vi "ToRepo.vi"(8 "error in":errorcluster, 9 "to repo cluster":T1, 10 "repository in":refnum<class "NISE_CEF_Repository.lvclass">, 11 "node in":refnum<class "NISE_CEF_serializable node.lvclass">) -> (0 "error out":errorcluster, 2 "repository out":refnum<class "NISE_CEF_Repository.lvclass">, 3 "node out":refnum<class "NISE_CEF_serializable node.lvclass">)   [LabVIEW 2013, in "NISE_CEF_serializable node.lvclass"]
doc: "Transfers the information from the tree node into the repo. How it is stored in the repo depends on the Repo."
uses:
  NISE_CEF_serializable node.lvclass
  Repository/NISE_CEF_Repository.lvclass
  Node/ToRepoCluster.ctl
  hierarchy repo/NISE_CEF_HierarchyRepo.lvclass
  Node/NISE_CEF_Node.lvclass
  serializable configuration/NISE_CEF_serializable configuration.lvclass/NISE_CEF_serializable configuration.ctl
  serializable configuration/NISE_CEF_serializable configuration.lvclass
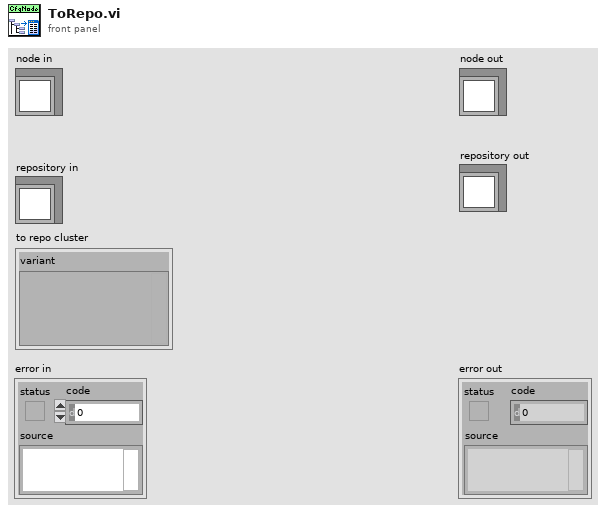
[diagram p1: front panel]
types:
  T1 = typedef "NISE_CEF_Node.lvclass/ToRepoCluster.ctl" = cluster{"variant":variant}
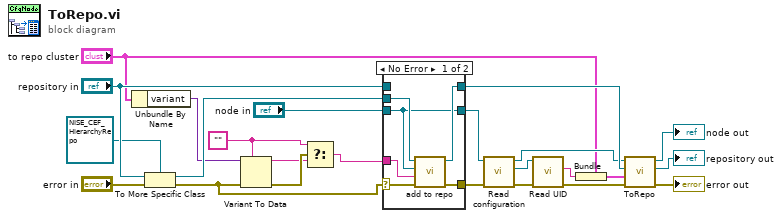
[diagram p0: block diagram]
diagram:
  w2 = ""
  n1 = Unbundle By Name("to repo cluster") -> ("variant"=w15:variant)
  n2 = To More Specific Class(target class=refnum<class "NISE_CEF_HierarchyRepo.lvclass"> refnum ("NISE_CEF_HierarchyRepo.lvclass"), reference="repository in", error in="error in") -> (specific class reference=w20:refnum<class "NISE_CEF_HierarchyRepo.lvclass">, error out=w5:errorcluster)
  n3 = Variant To Data(error in=w5, type=w2, Variant=w15) -> (data=w3:string, error out=w4:errorcluster)
  n4 = Select(t=w2, s=w4, f=w3) -> (s? t:f=w1:string)
  n5 = case shown="No Error" w5 {
    selector: w5 -> [w27 w32]
    tunnel: "repository in" -> [_ w33]
    tunnel: [w29 w33] -> w16
    tunnel: [w28 w32] -> w10
    tunnel: "node in" -> [w26 w31]
    tunnel: [w26 w31] -> w11
    tunnel: w20 -> [w30 _]
    tunnel: w1 -> [w25 _]
    frame No Error {
      n6 = call-dynamic "add to repo.vi"("error in"=w27, "parent"=w25, "serializable node"=w26, "NISE_CEF_HierarchyRepo in"=w30) -> ("error out"=w28:errorcluster, "NISE_CEF_HierarchyRepo out"=w29:refnum<class "NISE_CEF_HierarchyRepo.lvclass">)  [unwired: 6 in]
    }
    frame Error {
    }
  }
  n7 = call-dynamic "Read configuration.vi"("error in"=w10, "NISE_CEF_serializable node in"=w11) -> ("error out"=w9:errorcluster, "configuration"=w13:refnum<class "NISE_CEF_serializable configuration.lvclass">, "NISE_CEF_serializable node out"=w12:refnum<class "NISE_CEF_serializable node.lvclass">)  [unwired: 7 in]
  n8 = call "Read UID.vi"("error in"=w9, "configuration in"=w13) -> ("error out"=w14:errorcluster, "instance id"=w8:string)  [unwired: 7 in, 1 out]
  n9 = Bundle(cluster="to repo cluster", "variant"=w8) -> (w7:T1)
  n10 = call-parent "ToRepo.vi"("error in"=w14, "to repo cluster"=w7, "repository in"=w16, "node in"=w12) -> ("error out"=→"error out":errorcluster, "repository out"=→"repository out":refnum<class "NISE_CEF_Repository.lvclass">, "node out"=→"node out":refnum<class "NISE_CEF_serializable node.lvclass">)  [unwired: 5 in]
